vi "myRIO2.vi"() -> ()   [LabVIEW 2017]
uses:
  <vilib>/myRIO/Instrument Drivers/Onboard IO/DIO/typedefs/DIO Reference.ctl
  <vilib>/myRIO/Common/Instrument Driver Framework/Utilities/typedefs/myRIO Generic Hardware Reference.ctl
  <vilib>/myRIO/Common/Instrument Driver Framework/Utilities/typedefs/Hardware Version Enum.ctl
  <vilib>/myRIO/Common/Instrument Driver Framework/Utilities/typedefs/myRIO v1.0 Reference.ctl
  <vilib>/myRIO/Common/Instrument Driver Framework/Utilities/typedefs/Generic FPGA Reference.ctl
  <vilib>/myRIO/Common/Instrument Driver Framework/myRIO v1.0/DIO/typedefs/DIO Channels List.ctl
  <vilib>/myRIO/Common/Instrument Driver Framework/myRIO v1.0/DIO/typedefs/DIO Channels Enum.ctl
  <vilib>/userdefined/High Color/nirio_resource_hc.ctl
  <vilib>/Analysis/4window.llb/windowTd.ctl
  <vilib>/myRIO/Instrument Drivers/Onboard IO/UART/typedef/VISA Configuration.ctl
  <vilib>/myRIO/Common/Instrument Driver Framework/Utilities/vis/Is FPGA Ref Available.vi
  <vilib>/myRIO/Common/Instrument Driver Framework/myRIO v1.0/DIO/vis/myRIO v1.1 Open DIO.vi
  <vilib>/myRIO/Instrument Drivers/Onboard IO/DIO/vis/Write.vi
  <vilib>/myRIO/Instrument Drivers/Onboard IO/DIO/vis/Read.vi
  <vilib>/myRIO/Common/Instrument Driver Framework/Utilities/vis/Validate Channels.vi
  <vilib>/myRIO/Common/Instrument Driver Framework/myRIO v1.0/DIO/vis/myRIO v1.0 Reserve DIO.vi
  <vilib>/myRIO/Common/Instrument Driver Framework/myRIO v1.0/UART/vis/myRIO v1.0 Close UART.vi
  <vilib>/myRIO/Common/Instrument Driver Framework/myRIO v1.0/Resource Manager/vis/myRIO v1.0 Reserve Channel List.vi
  <vilib>/myRIO/Common/Instrument Driver Framework/myRIO v1.0/DIO/vis/myRIO v1.0 Build MUX Configuration DIO.vi
  <vilib>/myRIO/Common/Instrument Driver Framework/myRIO v1.0/Resource Manager/vis/myRIO v1.0 Reserve Channel.vi
  <vilib>/myRIO/Common/Instrument Driver Framework/myRIO v1.0/Resource Manager/vis/myRIO v1.0 Unreserve Channel.vi
  <vilib>/myRIO/Common/Instrument Driver Framework/myRIO v1.0/Resource Manager/vis/myRIO v1.0 Create Configuration List.vi
  <vilib>/myRIO/Common/Instrument Driver Framework/myRIO v1.0/Resource Manager/vis/myRIO v1.0 Build Mutex Name.vi
  <vilib>/Utility/VariantDataType/GetNumericInfo.vi
  <vilib>/Utility/error.llb/Error Cluster From Error Code.vi
  <vilib>/myRIO/Common/Instrument Driver Framework/myRIO v1.0/myRIO v1.1 Open.vi
  <vilib>/myRIO/Common/Instrument Driver Framework/Utilities/vis/IO Manager.vi
  <vilib>/myRIO/Common/Instrument Driver Framework/Utilities/vis/Configuration Manager.vi
  <vilib>/myRIO/Common/Instrument Driver Framework/myRIO v1.0/Resource Manager/vis/myRIO v1.0 Configure IO.vi
  <vilib>/myRIO/Common/Instrument Driver Framework/myRIO v1.0/myRIO v1.0 Close.vi
  <vilib>/myRIO/Common/Instrument Driver Framework/myRIO v1.0/DIO/vis/myRIO v1.0 Write DIO.vi
  <vilib>/FPGAPlugInAG/myRIO-1900/niLvFpga_Open_myRIO-1900.vi
  <vilib>/rvi/interface/common/dynamic/niFpgaDynamicAddResources.vi
  <vilib>/rvi/interface/common/niFpgaWaitOnOcc.vi
  <vilib>/rvi/errors/niLvFpgaAdjustHostInterfaceError.vi
  <vilib>/measure/maspectr.llb/FFT Power Spectrum and PSD for 1 Chan.vi
  <vilib>/FPGAPlugInAG/Dynamic/niLvFpga_Close_Dynamic.vi
  <vilib>/Instr/_visa.llb/VISA Configure Serial Port (Instr).vi
  <vilib>/myRIO/Common/Instrument Driver Framework/myRIO v1.0/DIO/vis/myRIO v1.0 Read DIO.vi
  <vilib>/Utility/file.llb/Write Delimited Spreadsheet (string).vi
  <vilib>/myRIO/Common/Instrument Driver Framework/Utilities/vis/FPGA Ref Manager.vi
  <vilib>/myRIO/Common/Instrument Driver Framework/myRIO v1.0/myRIO v1.0 Reset FPGA.vi
  <vilib>/myRIO/Common/Instrument Driver Framework/myRIO v1.0/IRQ/vis/myRIO v1.0 IRQ Info FGV.vi
  <vilib>/myRIO/Common/Instrument Driver Framework/myRIO v1.0/IRQ/vis/myRIO v1.0 Timer IRQ Info FGV.vi
  <vilib>/myRIO/Common/Instrument Driver Framework/myRIO v1.0/IRQ/vis/myRIO v1.0 ISR Agent.vi
  <vilib>/myRIO/Express VI/Onboard IO/DO/DO Express VI.xnode
  <vilib>/myRIO/Instrument Drivers/Onboard IO/DIO/vis/myRIO DIO Open.xnode
  <vilib>/rvi/interface/nirviOpenFPGA/nirviOpenFPGA.xnode
  drive-download-20180328T204708Z-001/Untitled Project 6/FPGA Bitfiles/UntitledProject6_FPGATarget_FPGA(1)_9+HZwm1Zn50.lvbitx
  FPGA (1).vi
  <vilib>/rvi/interface/nirviMethod/nirviMethod.xnode
  <vilib>/rvi/interface/nirviReadWriteControl/nirviReadWriteControl.xnode
  <vilib>/rvi/interface/nirviCloseFPGA/nirviCloseFPGA.xnode
  <vilib>/myRIO/Express VI/Onboard Devices/LED/LED Express VI.xnode
  <vilib>/myRIO/Express VI/Onboard IO/UART/UART Express VI.xnode
  <vilib>/myRIO/Express VI/Onboard IO/DI/DI Express VI.xnode
  <vilib>/myRIO/Express VI/Onboard Devices/Button/Button Express VI.xnode
  <vilib>/rvi/errors/niLvFpgaMergeErrorWithErrorCode.vi
  <vilib>/FPGAPlugInAG/Dynamic/niLvFpga_ReadFifo_Dynamic.vi
  <vilib>/FPGAPlugInAG/Dynamic/niLvFpga_ConfigureFifo_Dynamic.vi
  <vilib>/FPGAPlugInAG/Dynamic/niLvFpga_StartFifo_Dynamic.vi
  NiFpgaLv.dll
  <vilib>/rvi/interface/Simulation/niFpgaSimulationCallBeginRW.vi
  <vilib>/FPGAPlugInAG/Dynamic/niLvFpga_StopFifo_Dynamic.vi
  <vilib>/measure/NI_MAPro.lvlib
  <vilib>/myRIO/Instrument Drivers/Onboard IO/DIO/DIO.lvlib
  <vilib>/myRIO/Instrument Drivers/Onboard IO/UART/UART.lvlib
  <vilib>/myRIO/Instrument Drivers/Utilities/Utilities.lvlib
  <vilib>/Analysis/NI_AALPro.lvlib
panel:
  in  "Tab Control":enum32{"Logging  Data", "Amplitude Averaging"}(tab)
  out "Array 10":cluster{dbl, "y":dbl}[](array[cluster])
  out "Array 9":cluster{dbl, "y":dbl}[](array[cluster])
  out "Array 8":cluster{dbl, "y":dbl}[](array[cluster])
  out "Array 7":cluster{dbl, "y":dbl}[](array[cluster])
  out "Array 6":cluster{dbl, "y":dbl}[](array[cluster])
  out "element 2":cluster{dbl, "y":dbl}[](array[cluster])
  out "size":i32
  out "timed out?":bool
  out "# queue elements":i32
  out "Array 5":cluster{dbl, "y":dbl}[](array[cluster])
  in  "Array 4":cluster{dbl, "y":dbl}[](array[cluster])
  in  "Stop":bool
  out "Storage Device Failure":bool
  out "Data Queue Error":bool
  out "LinkIt Failure":bool
  out "DIO Failure":bool
  out "System Uptime":string
  out "Data Log Write Path":path
  out "Data Log":string[](array[string])
  out "D.L.H. Status":bool
  out "S.L.B. Status":bool
  out "D.L.B. Status":bool
  out "System Log Write Path":path
  out "System Log":string
  out "S.L.H. Status":bool
  out "Message Received":string
  out "M.R. Status":bool
  out "M.H. Status":bool
  out "LinkIt Response\nTimed Out 2":bool
  out "Time to Send \nMessage":dbl
  out "LinkIt Response\nTimed Out 3":bool
  out "LinkIt Response\nTimed Out 1":bool
  out "Pin 13 State":bool
  out "time to \nrespond":dbl
  out "Pin 11 State":bool
  out "Message to Send":string
  out "M.S. Status":bool
  out "?":i32(slide) scale=0.1..100.0
  out "S.L. Status":bool
  out "?":bool
  out "?":bool
  out "?":bool
  out "?":bool
  in  "Array 3":string[](array[string])
  out "Initialisation \nsuccessfull":bool
  in  "Min Frequency":dbl
  in  "Min Amplitude":dbl=0.001 format="%#_13g"
  out "Filtered Data Points":cluster{"X":dbl, "Y":dbl}[](graph)
  in  "averaging parameters":T1={"averaging mode"=enum."No averaging", "weighting mode"=enum."Exponential", "number of averages"=10} {"number of averages" min=1}
  out "Input Waveform":waveform(dbl)(graph)
  out "Power Spectrum":cluster{"f0":dbl, "df":dbl, "magnitude":dbl[]}(graph)
  out "error out":errorcluster
  out "Timed Out?":bool
  out "Maximum freq(Hz)":dbl
  out "Sampling freq(Hz)":dbl
  in  "Timeout (ms) 2":i32
  in  "No of Elements 2":u32=5000
  out "Element Read 2":i32
  out "Elements Remaining 2":u32
  out "Element Read":i32
  out "Current loop timing(ms)":u32
  in  "Count(uSec)":u32=16
  in  "Timeout (ms)":i32
  in  "No of Elements":u32
  out "Elements Remaining":u32
  in  "Requested Depth":u32=10000
  out "Actual Depth":u32=16384
  # "Project 2h - Version 1\nmyRIO1 Front Panel"
  # "FIFO configure"
  # "FPGA parameters"
  # "RT Loop Status"
  # "Signal Strength"
  # "Power Spectrum Options"
  # "Data point FIltering Options"
  # "FIFO Read"
  # "Outer"
  # "Inner"
  # "Rio \nDisplay"
  # "Elements to Read"
  # "Time out (ms)"
  # "Loop parameters"
  # "Elements Remaining"
  # "Elements Read"
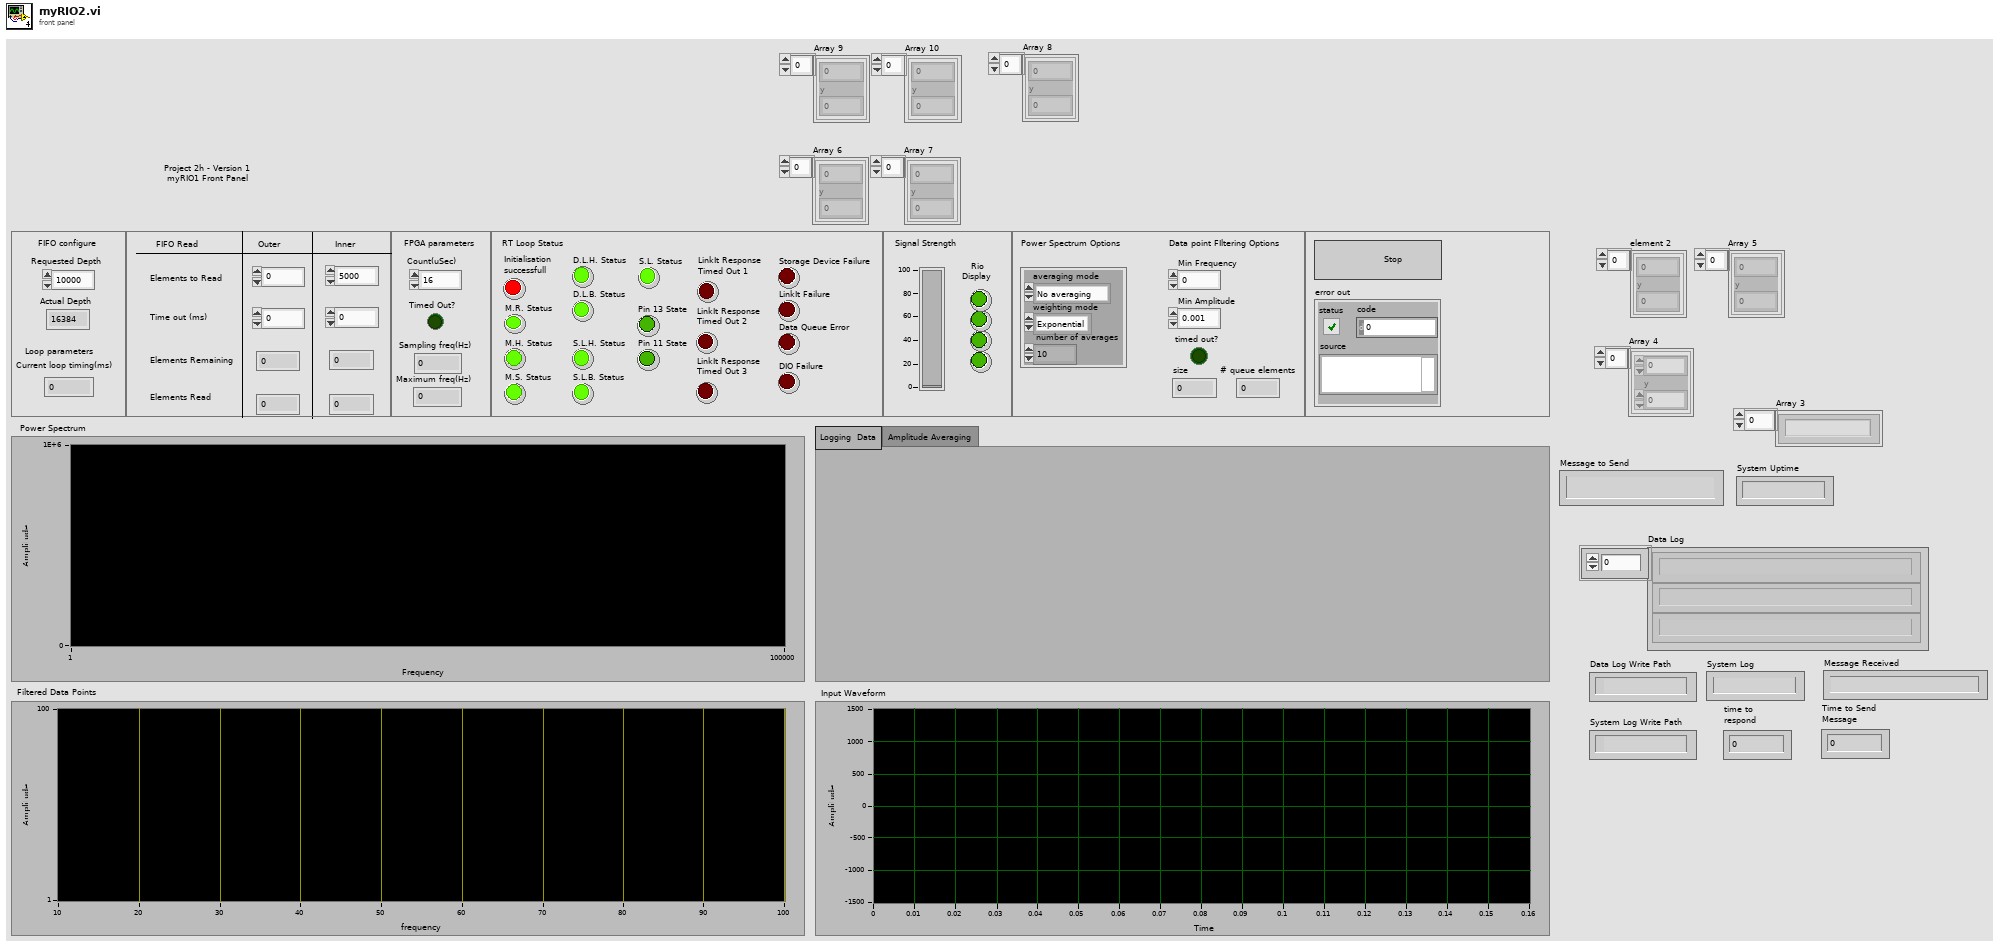
[diagram p1: front panel]
types:
  T1 = cluster{"averaging mode":enum16{"No averaging", "Vector averaging", "RMS averaging", "Peak hold"}, "weighting mode":enum16{"Linear", "Exponential"}, "number of averages":u32}
  T2 = cluster{string, string, string, string, string, string, string, string, string, string}
  T3 = typedef "DIO.lvlib/DIO Reference.ctl" = cluster{"myRIO Reference":T4, "DIO Channels List":T8}
  T4 = typedef "myRIO Generic Hardware Reference.ctl" = cluster{"myRIO Model":T5, "myRIO Hardware Reference":T6}
  T5 = typedef "Hardware Version Enum.ctl" = enum16{"Unknown", "myRIO-1900", "myRIO-1950", "roboRIO", "NI ELVIS RIO CM"}
  T6 = typedef "myRIO v1.0 Reference.ctl" = cluster{"Generic FPGA Reference":T7, "Allow multiple opens":bool}
  T7 = typedef "Generic FPGA Reference.ctl" = refnum<k20>
  T8 = typedef "DIO Channels List.ctl" = T9[]
  T9 = typedef "DIO Channels Enum.ctl" = enum16{"Not Connected", "C/DIO0", "C/DIO1", "C/DIO2", "C/DIO3", "C/DIO4", "C/DIO5", "C/DIO6", "C/DIO7", "A/DIO0", "A/DIO1", "A/DIO2", "A/DIO3", "A/DIO4", "A/DIO5", "A/DIO6", "A/DIO7", "A/DIO8", "A/DIO9", "A/DIO10", "A/DIO11", "A/DIO12", "A/DIO13", "A/DIO14", "A/DIO15", "B/DIO0", "B/DIO1", "B/DIO2", "B/DIO3", "B/DIO4", "B/DIO5", "B/DIO6", "B/DIO7", "B/DIO8", "B/DIO9", "B/DIO10", "B/DIO11", "B/DIO12", "B/DIO13", "B/DIO14", "B/DIO15", "LED0", "LED1", "LED2", "LED3", "Button0", "DIO/DIO0", "DIO/DIO1", "DIO/DIO2", "DIO/DIO3", "DIO/DIO4", "DIO/DIO5", "DIO/DIO6", "DIO/DIO7", "DIO/DIO8", "DIO/DIO9", "SPI/CS0", "SPI/CS1", "SPI/CS2", "SPI/CS3", "LED RADIO (Green)", "LED RADIO (Red)", "LED COMM (Green)", "LED COMM (Red)", "LED MODE (Green)", "LED MODE (Red)"}
  T10 = typedef "nirio_resource_hc.ctl" = tag
  T11 = typedef "UART.lvlib/VISA Configuration.ctl" = cluster{"baud rate (9600)":u32, "data bits (8)":u16, "parity (0:none)":enum16{"None", "Odd", "Even", "Mark", "Space"}, "stop bits (10: 1 bit)":u16, "flow control (0:none)":u16, "termination char\n(0xA = '\\n' = LF) ":u8, "Enable Termination\nChar (T)":bool, "timeout (10sec)":u32}
  T12 = enum16{"open", "replace", "create", "open or create", "replace or create", "replace or create with confirmation"}
  T13 = typedef "NI_AALPro.lvlib/windowTd.ctl" = u32
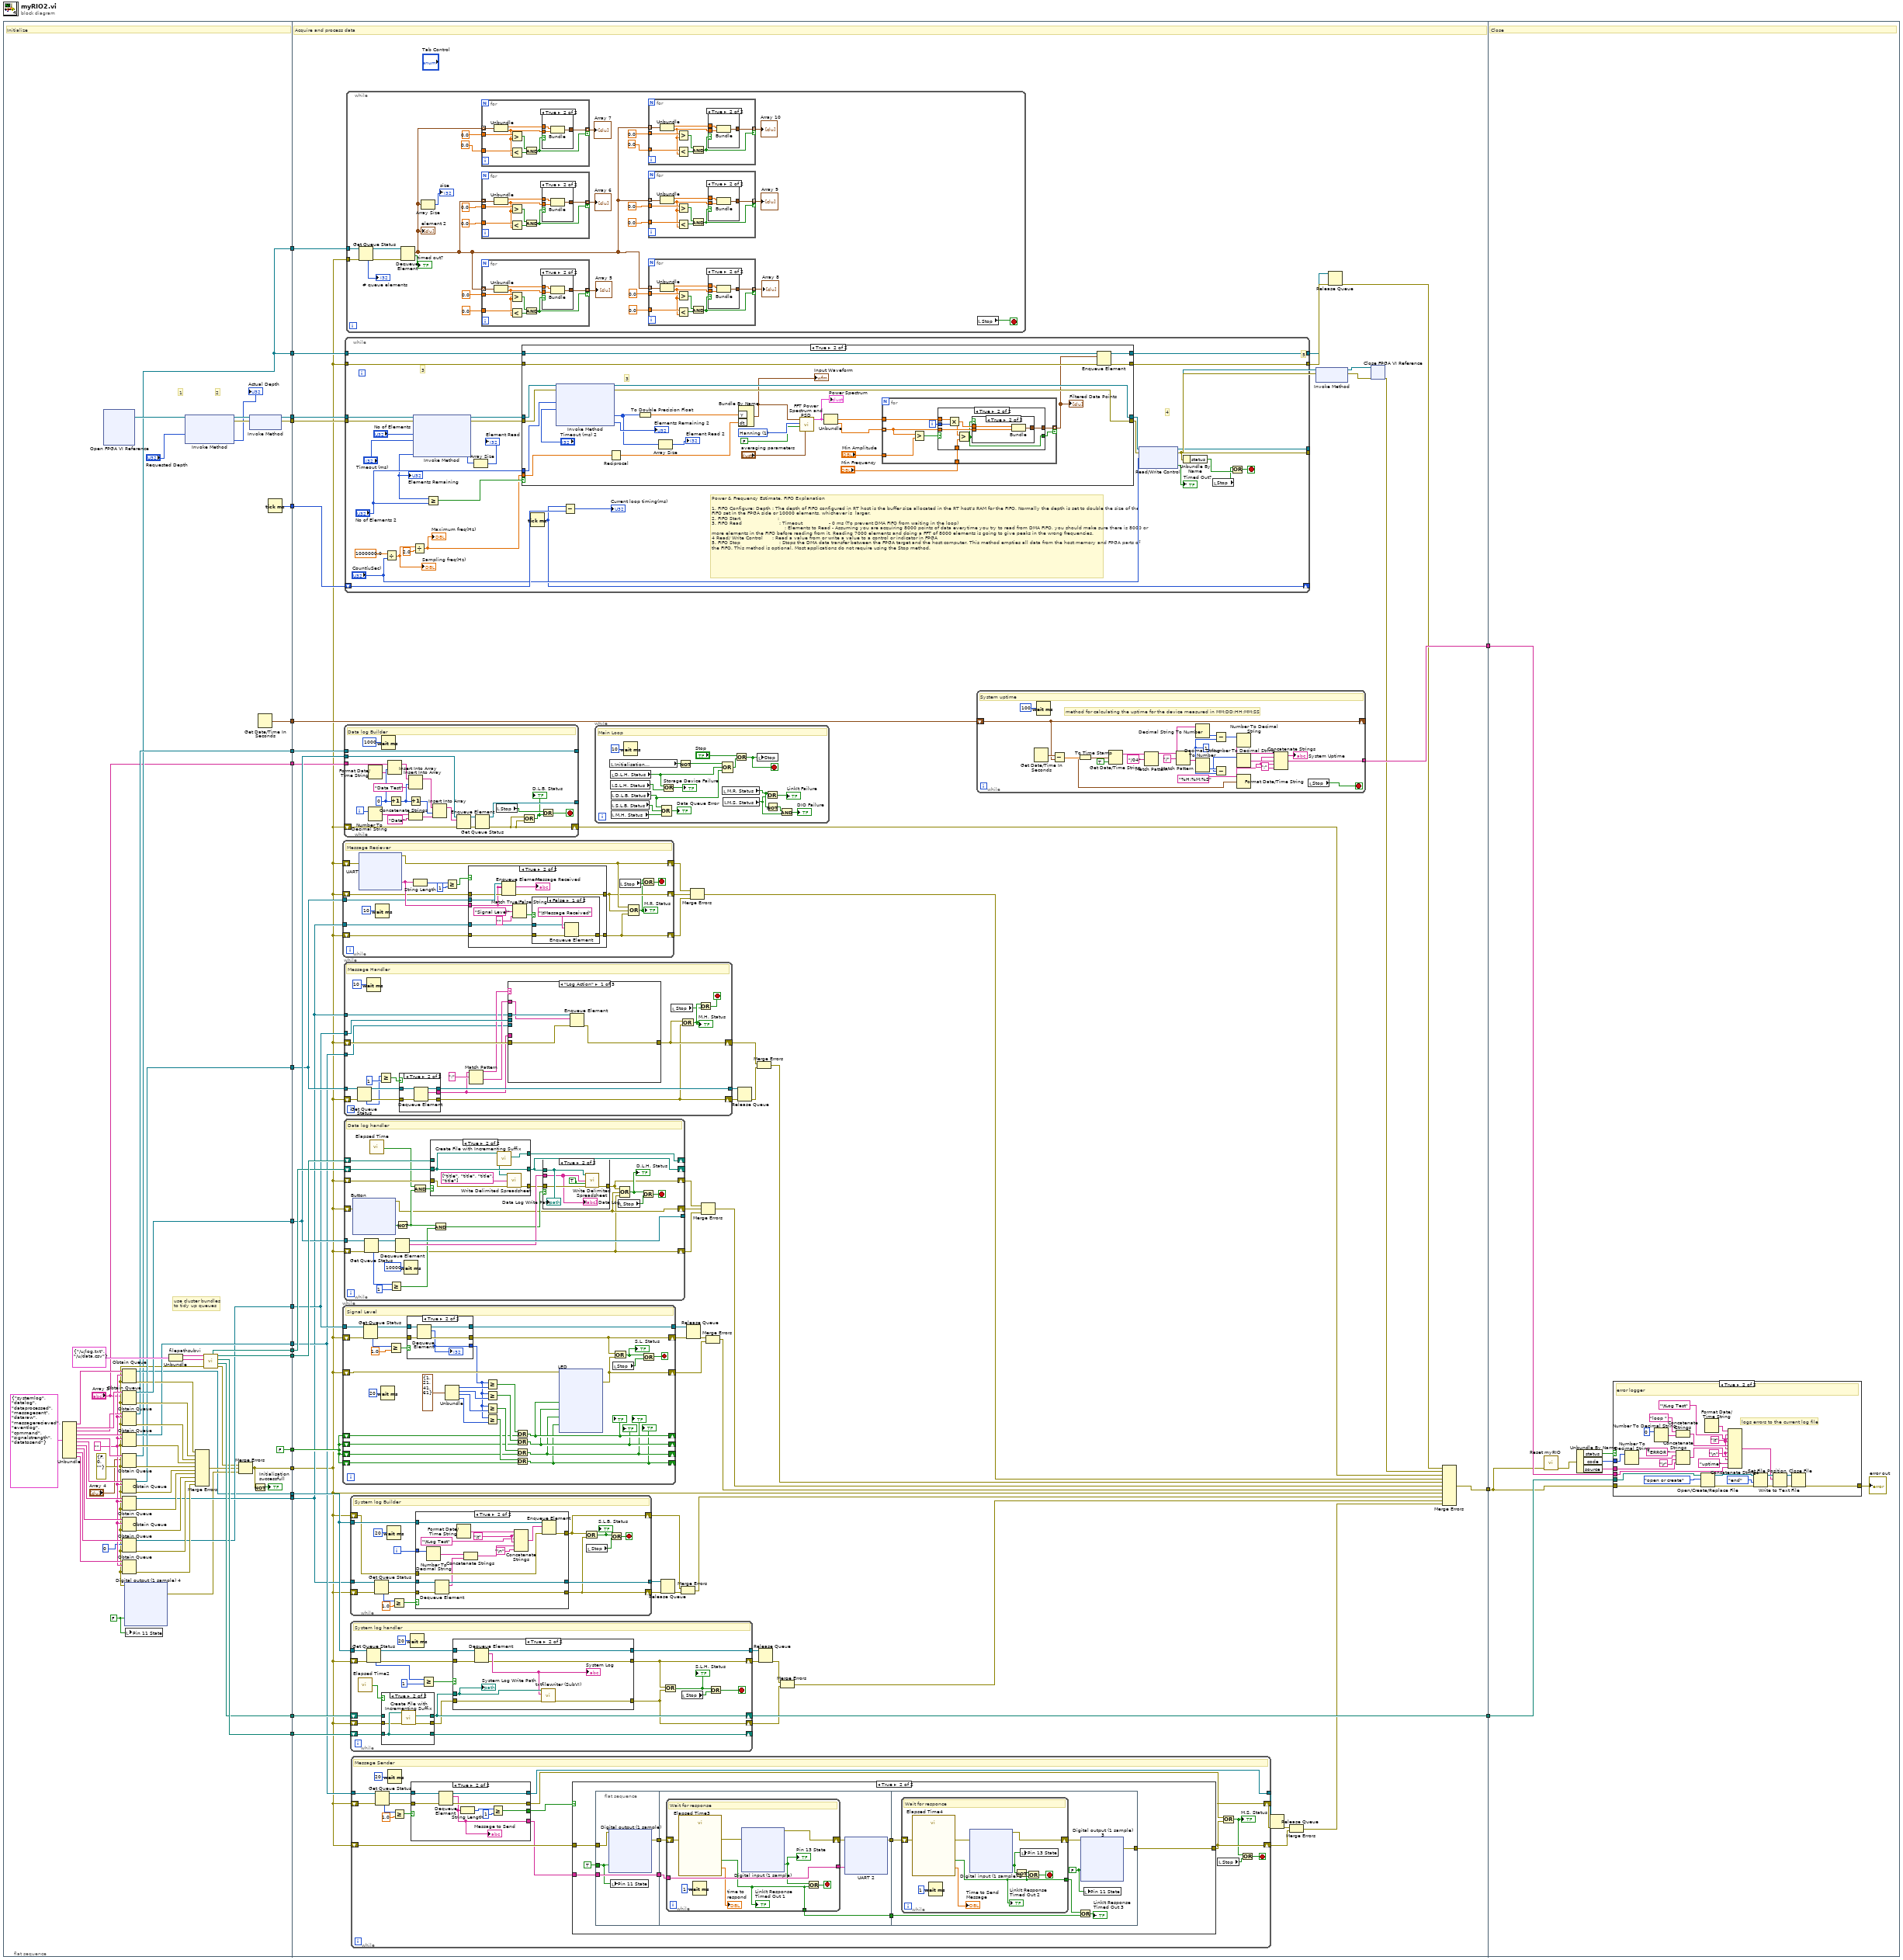
[diagram p0: block diagram]
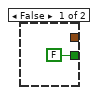
[diagram p9: hidden frame]
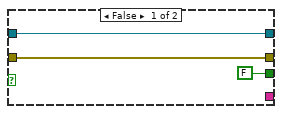
[diagram p12: hidden frame]
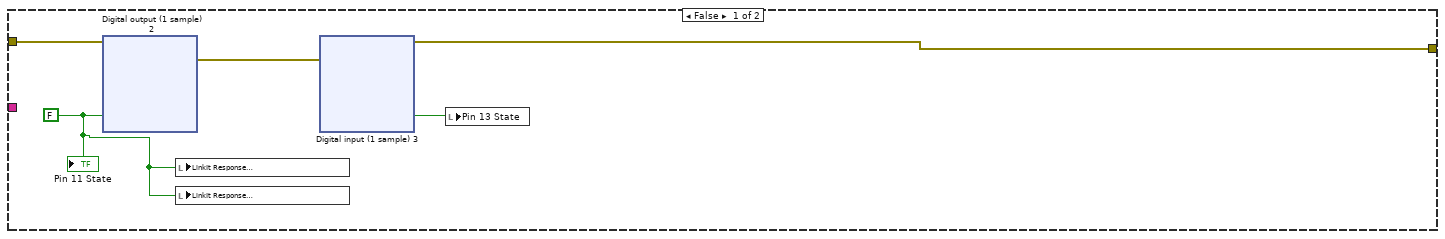
[diagram p13: hidden frame]
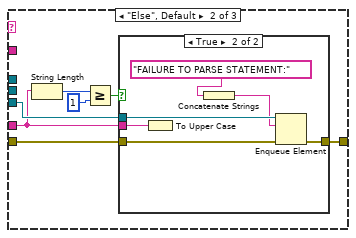
[diagram p15: hidden frame]
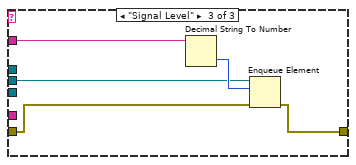
[diagram p17: hidden frame]
diagram:
  n1 = flat-sequence {
    tunnel: [w79] -> w23
    tunnel: [w70] -> w22
    tunnel: [w37] -> w21
    tunnel: [w69] -> w20
    tunnel: [w68] -> w19
    tunnel: [w35] -> w18
    tunnel: ["Array 3"] -> w17
    tunnel: [w36] -> w16
    tunnel: [w52] -> w15
    tunnel: [w51] -> w14
    tunnel: [w50] -> w13
    tunnel: [w49] -> w12
    tunnel: [w47] -> w11
    tunnel: [w46] -> w10
    tunnel: [FALSE] -> w9
    tunnel: [w29] -> w5
    tunnel: [w28] -> w4
    tunnel: [w27] -> w3
    tunnel: [w25] -> w2
    tunnel: [w25] -> w1
    tunnel: [w180] -> w8
    tunnel: w23 -> [w179]
    tunnel: w22 -> [w176]
    tunnel: w21 -> [w119]
    tunnel: w20 -> [w178]
    tunnel: w19 -> [w177]
    tunnel: w18 -> [w169]
    tunnel: w17 -> [w175]
    tunnel: w16 -> [w174]
    tunnel: w15 -> [w173]
    tunnel: w14 -> [w172]
    tunnel: [w171] -> w7
    tunnel: w13 -> [w170]
    tunnel: w12 -> [w141]
    tunnel: w11 -> [w131]
    tunnel: w10 -> [w144]
    tunnel: w9 -> [w166]
    tunnel: [w130] -> w6
    tunnel: w5 -> [w123]
    tunnel: w4 -> [w122]
    tunnel: w3 -> [w121]
    tunnel: w2 -> [w120]
    tunnel: w1 -> [w118]
    tunnel: w8 -> [w1064]
    tunnel: w7 -> [w1062]
    tunnel: w6 -> [w1061]
    frame #0 {
      w40 = FALSE
      w48 = ""
      w39 = errorcluster {"status"=FALSE, "code"=0, "source"=""} ("error in (no error)")
      # "2"
      # "1"
      # "use cluster bundles\nto tidy up queues"
      # "Initialize"
      n2 = Unbundle(T2 {"systemlog", "datalog", "dataprocessed", "messagesent", "dataraw", "messagerecieved", "eventlog", "command", "signalstrength", "datatosend"}) -> (w75:string, w74:string, w73:string, w72:string, w71:string, w62:string, w60:string, w59:string, w58:string, w57:string)
      n3 = xnode "Open FPGA VI Reference"() -> ("FPGA VI Reference Out"=w30:refnum<k20>)  [unwired: 2 in, 1 out]
      n4 = Obtain Queue(name (unnamed)=w75, element data type=w48, error in (no error)=w39) -> (queue out=w35:refnum<queue>, error out=w67:errorcluster)  [unwired: 2 in, 1 out]
      n5 = Obtain Queue(name (unnamed)=w74, element data type="Array 3", error in (no error)=w39) -> (queue out=w70:refnum<queue>, error out=w66:errorcluster)  [unwired: 2 in, 1 out]
      n6 = Obtain Queue(name (unnamed)=w73, element data type=w48, error in (no error)=w39) -> (queue out=w36:refnum<queue>, error out=w65:errorcluster)  [unwired: 2 in, 1 out]
      n7 = Obtain Queue(name (unnamed)=w72, element data type=w48, error in (no error)=w39) -> (queue out=w49:refnum<queue>, error out=w64:errorcluster)  [unwired: 2 in, 1 out]
      n8 = Obtain Queue(name (unnamed)=w71, element data type="Array 4", error in (no error)=w39) -> (queue out=w25:refnum<queue>, error out=w63:errorcluster)  [unwired: 2 in, 1 out]
      n9 = Obtain Queue(name (unnamed)=w62, element data type=w48, error in (no error)=w39) -> (queue out=w50:refnum<queue>, error out=w61:errorcluster)  [unwired: 2 in, 1 out]
      n10 = Obtain Queue(name (unnamed)=w60, element data type=w48, error in (no error)=w39) -> (queue out=w47:refnum<queue>, error out=w56:errorcluster)  [unwired: 2 in, 1 out]
      n11 = Obtain Queue(name (unnamed)=w59, element data type=w48, error in (no error)=w39) -> (error out=w55:errorcluster)  [unwired: 2 in, 2 out]
      n12 = Obtain Queue(name (unnamed)=w58, element data type=0, error in (no error)=w39) -> (queue out=w46:refnum<queue>, error out=w54:errorcluster)  [unwired: 2 in, 1 out]
      n13 = Obtain Queue(name (unnamed)=w57, element data type=w48, error in (no error)=w39) -> (error out=w53:errorcluster)  [unwired: 2 in, 2 out]
      n14 = xnode ("Digital output (1 sample) 4")("A/DIO0 (Pin 11)"=w40, "error in (no error)"=w39) -> ("error out"=w38:errorcluster)
      n15 = local write "Pin 11 State"(w40) -> ()
      n16 = Unbundle(cluster{string, string} {"/u/log.txt", "/u/data.csv"}) -> (w77:string, w76:string)
      n17 = xnode "Invoke Method"("FPGA VI Reference In"=w30, "Requested Depth"="Requested Depth") -> ("FPGA VI Reference Out"=w33:refnum<k20>, "error out"=w34:errorcluster, "Actual Depth"=→"Actual Depth":u32)  [unwired: 1 in]
      n18 = Merge Errors(w67, w66, w65, w64, w63, w61, w56, w55, w54, w53) -> (w42:errorcluster)
      n19 = call "filepathsubvi.vi"("error in (no error)"=w39, "String"=w76, "String 2"=w77) -> ("error out"=w41:errorcluster, "actual path"=w51:path, "Path"=w52:path, "actual path 2"=w69:path, "Path 2"=w68:path)  [unwired: 4 in]
      n20 = Merge Errors(w41, w42, w38) -> (w37:errorcluster)
      n21 = xnode "Invoke Method"("FPGA VI Reference In"=w33, "error in"=w34) -> ("FPGA VI Reference Out"=w28:refnum<k20>, "error out"=w27:errorcluster)
      n22 = Not(x=w37) -> (.not. x?=→"Initialisation \nsuccessfull":bool)
      n23 = Get Date/Time In Seconds() -> (seconds since 1Jan1904=w79:timestamp)
      n24 = Tick Count (ms)() -> (millisecond timer value=w29:u32)
    }
    frame #1 {
      # "5"
      # "Acquire and process data"
      n25 = while {
        shift-right: [w795] -> w151
        shift-left: w119 -> [w807]
        tunnel: w170 -> [w799]
        shift-right: [w794] -> w150
        shift-left: w119 -> [w798]
        shift-right: [w793] -> w149
        shift-left: w119 -> [w797]
        tunnel: w131 -> [w796]
        stop <- w804 stop-if-true
        # "Message Reciever"
        n26 = xnode "UART"("error in (no error)"=w807) -> ("Characters Read"=w800:string, "error out"=w795:errorcluster)
        n27 = Wait (ms)(milliseconds to wait=u32 10) -> ()  [unwired: 1 out]
        n28 = String Length(string=w800) -> (length=w802:i32)
        n29 = Greater Or Equal?(x=w802, y=1) -> (x >= y?=w803:bool)
        n30 = case shown="True" w803 {
          tunnel: w800 -> [_ w813]
          tunnel: w799 -> [_ w819]
          tunnel: w798 -> [w809 w818]
          tunnel: [w809 w817] -> w794
          tunnel: [w808 w816] -> w793
          tunnel: w797 -> [w808 w815]
          tunnel: w796 -> [_ w814]
          frame False {
          }
          frame True {
            n31 = Enqueue Element(queue=w819, element=w813, error in (no error)=w818) -> (error out=w817:errorcluster)  [unwired: 1 in, 2 out]
            n32 = Match True/False String(2:"" ("false string"), 3:"Signal Level" ("true string"), 4:w813) -> (0:w811:bool)  [unwired: 1 out]
            n33 = case shown="False" w811 {
              tunnel: [w822 w824] -> w816
              tunnel: w815 -> [w821 w824]
              tunnel: w814 -> [w820 _]
              frame False {
                n34 = Enqueue Element(queue=w820, element="\tMessage Received", error in (no error)=w821) -> (error out=w822:errorcluster)  [unwired: 1 in, 2 out]
              }
              frame True {
              }
            }
            "Message Received" <- w813
          }
        }
        n35 = local read "Stop"() -> (w805:bool)
        n36 = Compound Arithmetic op=OR(w795, w794, w793) -> (w792:bool)
        "M.R. Status" <- w792
        n37 = Or(x=w792, y=w805) -> (x .or. y?=w804:bool)
      }
      n38 = while {
        shift-right: [w365] -> w163
        shift-left: w119 -> [w376]
        shift-right: [w364] -> w154
        shift-left: w119 -> [w392]
        shift-right: [w369] -> _
        shift-left: w166 -> [w387]
        shift-right: [w368] -> _
        shift-left: w166 -> [w386]
        shift-right: [w367] -> _
        shift-left: w166 -> [w385]
        shift-right: [w366] -> _
        shift-left: w166 -> [w384]
        tunnel: w144 -> [w377]
        tunnel: [w375] -> w162
        stop <- w362 stop-if-true
        # "Signal Level"
        n39 = Get Queue Status(queue=w377, error in (no error)=w376) -> (queue out=w381:refnum<queue>, error out=w382:errorcluster, # elements in queue=w379:i32)  [unwired: 1 in, 5 out]
        n40 = Wait (ms)(milliseconds to wait=u32 20) -> ()  [unwired: 1 out]
        n41 = Greater Or Equal?(x=w379, y=1.0) -> (x >= y?=w380:bool)
        n42 = case shown="True" w380 {
          tunnel: w381 -> [w394 w399]
          tunnel: w382 -> [w393 w398]
          tunnel: [w394 w397] -> w375
          tunnel: [_ w395] -> w360
          tunnel: [w393 w396] -> w365
          frame False {
          }
          frame True {
            n43 = Dequeue Element(queue=w399, error in (no error)=w398) -> (queue out=w397:refnum<queue>, element=w395:i32, error out=w396:errorcluster)  [unwired: 1 in, 1 out]
            "?" <- w395
          }
        }
        n44 = Unbundle(cluster{i32, i32, i32, i32} {1, 21, 41, 61}) -> (w373:i32, w372:i32, w371:i32, w370:i32)
        n45 = Greater Or Equal?(x=w360, y=w373) -> (x >= y?=w391:bool)
        n46 = Greater Or Equal?(x=w360, y=w372) -> (x >= y?=w390:bool)
        n47 = Greater Or Equal?(x=w360, y=w371) -> (x >= y?=w389:bool)
        n48 = Greater Or Equal?(x=w360, y=w370) -> (x >= y?=w388:bool)
        n49 = Or(x=w391, y=w387) -> (x .or. y?=w369:bool)
        "?" <- w369
        n50 = Or(x=w390, y=w386) -> (x .or. y?=w368:bool)
        "?" <- w368
        n51 = Or(x=w389, y=w385) -> (x .or. y?=w367:bool)
        "?" <- w367
        n52 = Or(x=w388, y=w384) -> (x .or. y?=w366:bool)
        "?" <- w366
        n53 = xnode "LED"("61+"=w369, "41-60"=w368, "21-40"=w367, "1-20"=w366, "error in (no error)"=w392) -> ("error out"=w364:errorcluster)
        n54 = local read "Stop"() -> (w363:bool)
        n55 = Compound Arithmetic op=OR(w365, w364) -> (w361:bool)
        "S.L. Status" <- w361
        n56 = Or(x=w361, y=w363) -> (x .or. y?=w362:bool)
      }
      n57 = while {
        tunnel: [w760] -> w145
        tunnel: w170 -> [w759]
        shift-right: [w748] -> w146
        shift-left: w119 -> [w746]
        shift-right: [w753] -> w147
        shift-left: w119 -> [w757]
        tunnel: w144 -> [w756]
        tunnel: w141 -> [w749]
        tunnel: w131 -> [w740]
        stop <- w752 stop-if-true
        # "Message Handler"
        n58 = Get Queue Status(queue=w759, error in (no error)=w746) -> (queue out=w747:refnum<queue>, error out=w745:errorcluster, # elements in queue=w742:i32)  [unwired: 1 in, 5 out]
        n59 = Wait (ms)(milliseconds to wait=u32 10) -> ()  [unwired: 1 out]
        n60 = Greater Or Equal?(x=w742, y=1) -> (x >= y?=w743:bool)
        n61 = case shown="True" w743 {
          tunnel: [w763 w768] -> w760
          tunnel: [_ w767] -> w741
          tunnel: [w762 w766] -> w748
          tunnel: w747 -> [w763 w765]
          tunnel: w745 -> [w762 w764]
          frame False {
          }
          frame True {
            n62 = Dequeue Element(queue=w765, error in (no error)=w764) -> (queue out=w768:refnum<queue>, element=w767:string, error out=w766:errorcluster)  [unwired: 1 in, 1 out]
          }
        }
        n63 = Match Pattern(string=w741, regular expression=":") -> (before substring=w754:string, after substring=w755:string)  [unwired: 1 in, 2 out]
        n64 = case shown="\"Log Action\"" w754 {
          tunnel: w755 -> [w769 _ w790]
          tunnel: w757 -> [w772 w778 w789]
          tunnel: [w770 w777 w788] -> w753
          tunnel: w756 -> [_ _ w787]
          tunnel: w741 -> [_ w774 _]
          tunnel: w749 -> [_ w779 _]
          tunnel: w740 -> [w771 _ _]
          frame "Log Action" {
            n65 = Enqueue Element(queue=w771, element=w769, error in (no error)=w772) -> (error out=w770:errorcluster)  [unwired: 1 in, 2 out]
          }
          frame "Else", Default {
            n66 = String Length(string=w774) -> (length=w775:i32)
            n67 = Greater Or Equal?(x=w775, y=1) -> (x >= y?=w773:bool)
            n68 = case shown="True" w773 {
              tunnel: w779 -> [_ w786]
              tunnel: w778 -> [w780 w785]
              tunnel: [w780 w784] -> w777
              tunnel: w774 -> [_ w782]
              frame False {
              }
              frame True {
                n69 = To Upper Case(1:w782) -> ()  [unwired: 1 out]
                n70 = Concatenate Strings("FAILURE TO PARSE STATEMENT:") -> (w783:string)
                n71 = Enqueue Element(queue=w786, element=w783, error in (no error)=w785) -> (error out=w784:errorcluster)  [unwired: 1 in, 2 out]
              }
            }
          }
          frame "Signal Level" {
            n72 = Decimal String To Number(string=w790) -> (number=w791:i32)  [unwired: 2 in, 1 out]
            n73 = Enqueue Element(queue=w787, element=w791, error in (no error)=w789) -> (error out=w788:errorcluster)  [unwired: 1 in, 2 out]
          }
        }
        n74 = local read "Stop"() -> (w750:bool)
        n75 = Compound Arithmetic op=OR(w753, w748) -> (w751:bool)
        "M.H. Status" <- w751
        n76 = Or(x=w751, y=w750) -> (x .or. y?=w752:bool)
      }
      n77 = while {
        shift-right: [w959] -> w142
        shift-left: w119 -> [w955]
        tunnel: w176 -> [w967]
        tunnel: [w965] -> _
        shift-right: [w954] -> _
        shift-left: w177 -> [w953]
        shift-right: [w950] -> _
        shift-left: w178 -> [w951]
        shift-right: [w941] -> w148
        shift-left: w119 -> [w966]
        shift-right: [w942] -> w143
        shift-left: w119 -> [w943]
        stop <- w956 stop-if-true
        # "Data log handler"
        n78 = xnode "Button"("error in (no error)"=w943) -> ("Value"=w949:bool, "error out"=w942:errorcluster)
        n79 = Get Queue Status(queue=w967, error in (no error)=w966) -> (queue out=w964:refnum<queue>, error out=w963:errorcluster, # elements in queue=w962:i32)  [unwired: 1 in, 5 out]
        n80 = call "Elapsed Time"() -> ("Time has Elapsed"=w948:bool)  [unwired: 12 in, 7 out]
        n81 = Greater Or Equal?(x=w962, y=1) -> (x >= y?=w945:bool)
        n82 = Dequeue Element(queue=w964, error in (no error)=w963) -> (queue out=w965:refnum<queue>, element=w957:string[], error out=w941:errorcluster)  [unwired: 1 in, 1 out]
        n83 = Not(x=w949) -> (.not. x?=w946:bool)
        n84 = Wait (ms)(milliseconds to wait=u32 10000) -> ()  [unwired: 1 out]
        n85 = And(x=w948, y=w946) -> (x .and. y?=w947:bool)
        n86 = case shown="True" w947 {
          tunnel: w955 -> [w1005 w1011]
          tunnel: [w1006 w1008] -> w954
          tunnel: w953 -> [w1006 w1008]
          tunnel: [w1005 w1010] -> w952
          tunnel: w951 -> [w1004 _]
          tunnel: [w1004 w1007] -> w950
          frame False {
          }
          frame True {
            n87 = call <vilib>:"Create File with Incrementing Suffix.vi"("file path"=w1008) -> ("actual path"=w1007:path)  [unwired: 8 in, 2 out]
            n88 = call-poly <vilib>:"Write Delimited Spreadsheet.vi"("file path (dialog if empty)"=w1007, "1D data"=string[] ["title", "title", "title", "title"], "error in (no error)"=w1011) -> ("error out"=w1010:errorcluster)  [unwired: 11 in, 1 out]
          }
        }
        n89 = And(x=w946, y=w945) -> (x .and. y?=w944:bool)
        n90 = case shown="True" w944 {
          tunnel: w952 -> [w1012 w1016]
          tunnel: w954 -> [_ w1017]
          tunnel: [w1012 w1015] -> w959
          tunnel: w957 -> [_ w1013]
          frame False {
          }
          frame True {
            n91 = call-poly <vilib>:"Write Delimited Spreadsheet.vi"("file path (dialog if empty)"=w1017, "1D data"=w1013, "append to file? (new file:F)"=TRUE, "error in (no error)"=w1016) -> ("error out"=w1015:errorcluster)  [unwired: 10 in, 1 out]
            "Data Log Write Path" <- w1017
            "Data Log" <- w1013
          }
        }
        n92 = local read "Stop"() -> (w958:bool)
        n93 = Compound Arithmetic op=OR(w959, w942, w941) -> (w960:bool)
        "D.L.H. Status" <- w960
        n94 = Or(x=w960, y=w958) -> (x .or. y?=w956:bool)
      }
      n95 = while {
        tunnel: w176 -> [w903]
        tunnel: [w900] -> _
        tunnel: [w884] -> _
        tunnel: w174 -> [w884]
        tunnel: w175 -> [w883]
        shift-right: [w882] -> w139
        shift-left: w119 -> [w899]
        i -> [w887]
        stop <- w886 stop-if-true
        w895 = 0
        # "Data log Builder"
        n96 = Format Date/Time String() -> (date/time string=w892:string)  [unwired: 3 in]
        n97 = Number To Decimal String(number=w887) -> (decimal integer string=w890:string)  [unwired: 1 in]
        n98 = Wait (ms)(milliseconds to wait=u32 1000) -> ()  [unwired: 1 out]
        n99 = Insert Into Array(array=w883, index=w895, new element=w892) -> (w898:string[])
        n100 = Increment(x=w895) -> (x+1=w894:i32)
        n101 = Concatenate Strings(w890, "Data") -> (w888:string)
        n102 = Insert Into Array(array=w898, index=w894, new element="Data Test" ("text")) -> (w897:string[])
        n103 = Increment(x=w894) -> (x+1=w893:i32)
        n104 = Insert Into Array(array=w897, index=w893, new element=w888) -> (w896:string[])
        n105 = Enqueue Element(queue=w903, element=w896, error in (no error)=w899) -> (queue out=w901:refnum<queue>, error out=w902:errorcluster)  [unwired: 1 in, 1 out]
        n106 = Get Queue Status(queue=w901, error in (no error)=w902) -> (queue out=w900:refnum<queue>, error out=w882:errorcluster)  [unwired: 1 in, 6 out]
        n107 = local read "Stop"() -> (w885:bool)
        n108 = Compound Arithmetic op=OR(w882, w882) -> (w881:bool)
        "D.L.B. Status" <- w881
        n109 = Or(x=w885, y=w881) -> (x .or. y?=w886:bool)
      }
      n110 = while {
        tunnel: w122 -> [w310]
        tunnel: w121 -> [w309]
        tunnel: [w305] -> w124
        tunnel: [w288] -> w125
        shift-right: [w289] -> _
        shift-left: w123 -> [w303]
        tunnel: w120 -> [w286]
        tunnel: [w285] -> w128
        tunnel: w119 -> [w284]
        tunnel: [w283] -> w129
        stop <- w306 stop-if-true
        # "Power & Frequency Estimate. FIFO Explanation\n\n1. FIFO Configure: Depth : The depth of FIFO configured in RT host is the buffer size allocated in the RT host's RAM for the FIFO. Normally the depth is set to double the size of the FIFO set in the FPGA side or 10000 elements, whichever is  larger.\n2. FIFO Start                        :\n3. FIFO Read                        : Timeout                 - 0 ms (To prevent DMA FIFO from waiting in the loop) \n                                               : Elements to Read - Assuming you are acquiring 8000 points of data everytime you try to read from DMA FIFO, you should make sure there is 8000 or more elements in the FIFO before reading from it. Reading 7000 elements and doing a FFT of 8000 elements is going to give peaks in the wrong frequencies.\n4 Read/ Write Control      : Read a value from or write a value to a control or indicator in FPGA \n5. FIFO Stop                         : Stops the DMA data transfer between the FPGA target and the host computer. This method empties all data from the host memory and FPGA parts of the FIFO. This method is optional. Most applications do not require using the Stop method."
        # "4"
        # "3"
        n111 = Divide(x=1000000.0 ("y"), y="Count(uSec)") -> (x/y=w282:dbl)
        "Sampling freq(Hz)" <- w282
        n112 = Divide(x=w282, y=2.0) -> (x/y=w281:dbl)
        "Maximum freq(Hz)" <- w281
        n113 = xnode "Invoke Method"("FPGA VI Reference In"=w310, "error in"=w309, "Number of Elements"="No of Elements", "Timeout (ms)"="Timeout (ms)") -> ("FPGA VI Reference Out"=w297:refnum<k20>, "error out"=w296:errorcluster, "Data"=w301:i16[], "Elements Remaining"=w299:u32)
        "Elements Remaining" <- w299
        n114 = Greater Or Equal?(x=w299, y="No of Elements 2") -> (x >= y?=w298:bool)
        n115 = Array Size(array=w301) -> (size(s)=→"Element Read":i32)
        n116 = case shown="True" w298 {
          tunnel: "No of Elements 2" -> [_ w340]
          tunnel: w297 -> [w314 w339]
          tunnel: w296 -> [w313 w338]
          tunnel: [w314 w337] -> w295
          tunnel: [w313 w330] -> w294
          tunnel: w286 -> [w311 w327]
          tunnel: [w311 w326] -> w285
          tunnel: w284 -> [w312 w325]
          tunnel: [w312 w324] -> w283
          tunnel: w281 -> [_ w321]
          frame False {
          }
          frame True {
            w333 = T13 1 items=["Rectangle"=0, "Hanning"=1, "Hamming"=2, "Blackman-Harris"=3, "Exact Blackman"=4, "Blackman"=5, "Flat Top"=6, "4 Term B-Harris "=7, "7 Term B-Harris"=8, "Low Sidelobe"=9, "Blackman Nuttall"=11, "Triangle"=30, "Bartlett-Hanning"=31, "Bohman"=32, "Parzen"=33, "Welch"=34, "Kaiser"=60, "Dolph-Chebyshev"=61, "Gaussian"=62] ("window")
            # "3"
            n117 = xnode "Invoke Method"("FPGA VI Reference In"=w339, "error in"=w338, "Number of Elements"=w340, "Timeout (ms)"="Timeout (ms) 2") -> ("FPGA VI Reference Out"=w337:refnum<k20>, "error out"=w330:errorcluster, "Data"=w331:i16[], "Elements Remaining"=→"Elements Remaining 2":u32)
            n118 = Reciprocal(x=w321) -> (1/x=w329:dbl)
            n119 = To Double Precision Float(number=w331) -> (double precision float=w322:dbl[])
            n120 = Array Size(array=w331) -> (size(s)=→"Element Read 2":i32)
            n121 = Bundle By Name("Y"=w322, "dt"=w329) -> (w323:waveform(dbl))  [unwired: 1 in]
            "Input Waveform" <- w323
            n122 = call-poly <vilib>:"FFT Power Spectrum and PSD.vi"("averaging parameters"="averaging parameters", "dB On (F)"=FALSE, "window"=w333, "time signal"=w323) -> ("Power Spectrum / PSD"=w320:cluster{"f0":dbl, "df":dbl, "magnitude":dbl[]})  [unwired: 4 in, 3 out]
            "Power Spectrum" <- w320
            n123 = Unbundle(w320) -> ("df"=w319:dbl, "magnitude"=w316:dbl[])  [unwired: 1 out]
            n124 = for {
              tunnel: w316 -> [w346] mode=indexing
              tunnel: w319 -> [w348]
              tunnel: [w345] -> w315 mode=indexing if=w341
              tunnel: "Min Amplitude" -> [w344]
              tunnel: "Min Frequency" -> [w343]
              i -> [w347]
              n125 = Greater?(x=w346, y=w344) -> (0:w342:bool)
              n126 = case shown="True" w342 {
                tunnel: w348 -> [_ w356]
                tunnel: w347 -> [_ w353]
                tunnel: w346 -> [_ w354]
                tunnel: [_ w355] -> w345
                tunnel: w343 -> [_ w351]
                tunnel: [FALSE w350] -> w341
                frame False {
                }
                frame True {
                  n127 = Multiply(x=w356, y=w353) -> (x*y=w352:dbl)
                  n128 = Greater?(x=w352, y=w351) -> (0:w350:bool)
                  n129 = case shown="True" w350 {
                    tunnel: [_ w359] -> w355
                    tunnel: w352 -> [_ w358]
                    tunnel: w354 -> [_ w357]
                    frame False {
                    }
                    frame True {
                      n130 = Bundle(w358, "Numeric"=w357) -> (w359:cluster{dbl, "Numeric":dbl})  [unwired: 1 in]
                    }
                  }
                }
              }
            }
            "Filtered Data Points" <- w315
            n131 = Enqueue Element(queue=w327, element=w315, error in (no error)=w325) -> (queue out=w326:refnum<queue>, error out=w324:errorcluster)  [unwired: 1 in, 1 out]
          }
        }
        n132 = Tick Count (ms)() -> (millisecond timer value=w289:u32)
        n133 = Subtract(x=w289, y=w303) -> (x-y=→"Current loop timing(ms)":u32)
        n134 = xnode "Read/Write Control"("FPGA VI Reference In"=w295, "error in"=w294, "Count(uSec)"="Count(uSec)") -> ("FPGA VI Reference Out"=w305:refnum<k20>, "error out"=w288:errorcluster, "Timed Out?"=→"Timed Out?":bool)
        n135 = Unbundle By Name(w288) -> ("status"=w287:bool)
        n136 = local read "Stop"() -> (w280:bool)
        n137 = Or(x=w280, y=w287) -> (x .or. y?=w306:bool)
      }
      n138 = while {
        tunnel: w118 -> [w205]
        tunnel: w119 -> [w203]
        stop <- w191 stop-if-true
        n139 = Get Queue Status(queue=w205, error in (no error)=w203) -> (queue out=w204:refnum<queue>, error out=w202:errorcluster, # elements in queue=→"# queue elements":i32)  [unwired: 1 in, 5 out]
        n140 = Dequeue Element(queue=w204, error in (no error)=w202) -> (element=w181:cluster{dbl, "y":dbl}[], timed out?=→"timed out?":bool)  [unwired: 1 in, 2 out]
        "element 2" <- w181
        n141 = Array Size(array=w181) -> (size(s)=→"size":i32)
        n142 = for {
          tunnel: w181 -> [w252] mode=indexing
          tunnel: 0.0 -> [w251]
          tunnel: 0.0 -> [w250]
          tunnel: [w245] -> w193 mode=indexing if=w244
          n143 = Unbundle(w252) -> (w247:dbl, "y"=w246:dbl)
          n144 = Greater?(x=w250, y=w246) -> (0:w249:bool)
          n145 = Less?(x=w251, y=w246) -> (x < y?=w248:bool)
          n146 = And(x=w249, y=w248) -> (x .and. y?=w244:bool)
          n147 = case shown="True" w244 {
            tunnel: w247 -> [_ w255]
            tunnel: w246 -> [_ w254]
            tunnel: [_ w253] -> w245
            frame False {
            }
            frame True {
              n148 = Bundle(w255, "y"=w254) -> (w253:cluster{dbl, "y":dbl})  [unwired: 1 in]
            }
          }
        }
        "Array 7" <- w193
        n149 = for {
          tunnel: w181 -> [w264] mode=indexing
          tunnel: 0.0 -> [w263]
          tunnel: 0.0 -> [w262]
          tunnel: [w257] -> w192 mode=indexing if=w256
          n150 = Unbundle(w264) -> (w259:dbl, "y"=w258:dbl)
          n151 = Greater?(x=w262, y=w258) -> (0:w261:bool)
          n152 = Less?(x=w263, y=w258) -> (x < y?=w260:bool)
          n153 = And(x=w261, y=w260) -> (x .and. y?=w256:bool)
          n154 = case shown="True" w256 {
            tunnel: w259 -> [_ w267]
            tunnel: w258 -> [_ w266]
            tunnel: [_ w265] -> w257
            frame False {
            }
            frame True {
              n155 = Bundle(w267, "y"=w266) -> (w265:cluster{dbl, "y":dbl})  [unwired: 1 in]
            }
          }
        }
        "Array 6" <- w192
        n156 = for {
          tunnel: w181 -> [w276] mode=indexing
          tunnel: 0.0 -> [w275]
          tunnel: 0.0 -> [w274]
          tunnel: [w269] -> w198 mode=indexing if=w268
          n157 = Unbundle(w276) -> (w271:dbl, "y"=w270:dbl)
          n158 = Greater?(x=w274, y=w270) -> (0:w273:bool)
          n159 = Less?(x=w275, y=w270) -> (x < y?=w272:bool)
          n160 = And(x=w273, y=w272) -> (x .and. y?=w268:bool)
          n161 = case shown="True" w268 {
            tunnel: w271 -> [_ w279]
            tunnel: w270 -> [_ w278]
            tunnel: [_ w277] -> w269
            frame False {
            }
            frame True {
              n162 = Bundle(w279, "y"=w278) -> (w277:cluster{dbl, "y":dbl})  [unwired: 1 in]
            }
          }
        }
        "Array 5" <- w198
        n163 = for {
          tunnel: w181 -> [w216] mode=indexing
          tunnel: 0.0 -> [w215]
          tunnel: 0.0 -> [w214]
          tunnel: [w209] -> w183 mode=indexing if=w208
          n164 = Unbundle(w216) -> (w211:dbl, "y"=w210:dbl)
          n165 = Greater?(x=w214, y=w210) -> (0:w213:bool)
          n166 = Less?(x=w215, y=w210) -> (x < y?=w212:bool)
          n167 = And(x=w213, y=w212) -> (x .and. y?=w208:bool)
          n168 = case shown="True" w208 {
            tunnel: w211 -> [_ w219]
            tunnel: w210 -> [_ w218]
            tunnel: [_ w217] -> w209
            frame False {
            }
            frame True {
              n169 = Bundle(w219, "y"=w218) -> (w217:cluster{dbl, "y":dbl})  [unwired: 1 in]
            }
          }
        }
        "Array 10" <- w183
        n170 = for {
          tunnel: w181 -> [w228] mode=indexing
          tunnel: 0.0 -> [w227]
          tunnel: 0.0 -> [w226]
          tunnel: [w221] -> w182 mode=indexing if=w220
          n171 = Unbundle(w228) -> (w223:dbl, "y"=w222:dbl)
          n172 = Greater?(x=w226, y=w222) -> (0:w225:bool)
          n173 = Less?(x=w227, y=w222) -> (x < y?=w224:bool)
          n174 = And(x=w225, y=w224) -> (x .and. y?=w220:bool)
          n175 = case shown="True" w220 {
            tunnel: w223 -> [_ w231]
            tunnel: w222 -> [_ w230]
            tunnel: [_ w229] -> w221
            frame False {
            }
            frame True {
              n176 = Bundle(w231, "y"=w230) -> (w229:cluster{dbl, "y":dbl})  [unwired: 1 in]
            }
          }
        }
        "Array 9" <- w182
        n177 = for {
          tunnel: w181 -> [w240] mode=indexing
          tunnel: 0.0 -> [w239]
          tunnel: 0.0 -> [w238]
          tunnel: [w233] -> w188 mode=indexing if=w232
          n178 = Unbundle(w240) -> (w235:dbl, "y"=w234:dbl)
          n179 = Greater?(x=w238, y=w234) -> (0:w237:bool)
          n180 = Less?(x=w239, y=w234) -> (x < y?=w236:bool)
          n181 = And(x=w237, y=w236) -> (x .and. y?=w232:bool)
          n182 = case shown="True" w232 {
            tunnel: w235 -> [_ w243]
            tunnel: w234 -> [_ w242]
            tunnel: [_ w241] -> w233
            frame False {
            }
            frame True {
              n183 = Bundle(w243, "y"=w242) -> (w241:cluster{dbl, "y":dbl})  [unwired: 1 in]
            }
          }
        }
        "Array 8" <- w188
        n184 = local read "Stop"() -> (w191:bool)
      }
      n185 = while {
        shift-right: [w908] -> w158
        shift-left: w119 -> [w909]
        tunnel: w131 -> [w914]
        tunnel: [w912] -> w168
        shift-right: [w907] -> w167
        shift-left: w119 -> [w913]
        tunnel: w169 -> [w910]
        i -> [w905]
        stop <- w919 stop-if-true
        # "System log Builder"
        n186 = Get Queue Status(queue=w914, error in (no error)=w913) -> (queue out=w916:refnum<queue>, error out=w915:errorcluster, # elements in queue=w918:i32)  [unwired: 1 in, 5 out]
        n187 = Wait (ms)(milliseconds to wait=u32 20) -> ()  [unwired: 1 out]
        n188 = Greater Or Equal?(x=w918, y=1.0) -> (x >= y?=w911:bool)
        n189 = case shown="True" w911 {
          tunnel: w916 -> [w923 w940]
          tunnel: w915 -> [w924 w939]
          tunnel: [w923 w938] -> w912
          tunnel: [w924 w937] -> w907
          tunnel: w905 -> [_ w930]
          tunnel: w910 -> [_ w929]
          tunnel: w909 -> [w922 w927]
          tunnel: [w922 w925] -> w908
          frame False {
          }
          frame True {
            w933 = "\t"
            n190 = Number To Decimal String(number=w930) -> (decimal integer string=w934:string)  [unwired: 1 in]
            n191 = Dequeue Element(queue=w940, error in (no error)=w939) -> (queue out=w938:refnum<queue>, element=w926:string, error out=w937:errorcluster)  [unwired: 1 in, 1 out]
            n192 = Format Date/Time String() -> (date/time string=w935:string)  [unwired: 3 in]
            n193 = Concatenate Strings(w934, w926) -> (w936:string)
            n194 = Concatenate Strings(w935, w933, "\tLog Test" ("text"), w933, w936, "\n") -> (w928:string)
            n195 = Enqueue Element(queue=w929, element=w928, error in (no error)=w927) -> (error out=w925:errorcluster)  [unwired: 1 in, 2 out]
          }
        }
        n196 = Compound Arithmetic op=OR(w908, w907) -> (w906:bool)
        "S.L.B. Status" <- w906
        n197 = local read "Stop"() -> (w920:bool)
        n198 = Or(x=w906, y=w920) -> (x .or. y?=w919:bool)
      }
      n199 = while {
        shift-right: [w844] -> w157
        shift-left: w119 -> [w848]
        tunnel: w169 -> [w861]
        shift-right: [w850] -> w171
        shift-left: w172 -> [w852]
        shift-right: [w849] -> _
        shift-left: w173 -> [w851]
        shift-right: [w843] -> w160
        shift-left: w119 -> [w860]
        tunnel: [w842] -> w161
        stop <- w854 stop-if-true
        # "System log handler"
        n200 = call "Elapsed Time2"() -> ("Time has Elapsed"=w853:bool)  [unwired: 12 in, 7 out]
        n201 = Get Queue Status(queue=w861, error in (no error)=w860) -> (queue out=w846:refnum<queue>, error out=w845:errorcluster, # elements in queue=w859:i32)  [unwired: 1 in, 5 out]
        n202 = case shown="True" w853 {
          tunnel: w851 -> [w865 w868]
          tunnel: [w864 w869] -> w850
          tunnel: [w865 w868] -> w849
          tunnel: w852 -> [w864 _]
          tunnel: w848 -> [w863 w867]
          tunnel: [w863 w866] -> w847
          frame False {
          }
          frame True {
            n203 = call <vilib>:"Create File with Incrementing Suffix.vi"("error in (no error)"=w867, "file path"=w868) -> ("error out"=w866:errorcluster, "actual path"=w869:path)  [unwired: 7 in, 1 out]
          }
        }
        n204 = Wait (ms)(milliseconds to wait=u32 20) -> ()  [unwired: 1 out]
        n205 = Greater Or Equal?(x=w859, y=1) -> (x >= y?=w857:bool)
        n206 = case shown="True" w857 {
          tunnel: w847 -> [w872 w880]
          tunnel: w850 -> [_ w879]
          tunnel: [w872 w878] -> w844
          tunnel: w846 -> [w870 w877]
          tunnel: w845 -> [w871 w876]
          tunnel: [w871 w874] -> w843
          tunnel: [w870 w873] -> w842
          frame False {
          }
          frame True {
            n207 = Dequeue Element(queue=w877, error in (no error)=w876) -> (queue out=w873:refnum<queue>, element=w875:string, error out=w874:errorcluster)  [unwired: 1 in, 1 out]
            "System Log" <- w875
            n208 = call "txtfilewriter (SubVI).vi"("error in (no error)"=w880, "String"=w875, "actual path"=w879) -> ("error out"=w878:errorcluster)  [unwired: 8 in]
            "System Log Write Path" <- w879
          }
        }
        n209 = Compound Arithmetic op=OR(w843, w844) -> (w856:bool)
        "S.L.H. Status" <- w856
        n210 = local read "Stop"() -> (w855:bool)
        n211 = Or(x=w856, y=w855) -> (x .or. y?=w854:bool)
      }
      n212 = while {
        shift-right: [w442] -> w152
        shift-left: w119 -> [w454]
        tunnel: w141 -> [w445]
        tunnel: [w449] -> w165
        shift-right: [w441] -> w164
        shift-left: w119 -> [w444]
        stop <- w438 stop-if-true
        # "Message Sender"
        n213 = Get Queue Status(queue=w445, error in (no error)=w444) -> (queue out=w446:refnum<queue>, error out=w443:errorcluster, # elements in queue=w451:i32)  [unwired: 1 in, 5 out]
        n214 = Wait (ms)(milliseconds to wait=u32 20) -> ()  [unwired: 1 out]
        n215 = Greater Or Equal?(x=w451, y=1.0) -> (x >= y?=w447:bool)
        n216 = case shown="True" w447 {
          tunnel: w446 -> [w457 w463]
          tunnel: w443 -> [w456 w462]
          tunnel: [FALSE w461] -> w450
          tunnel: [w457 w460] -> w449
          tunnel: [_ w458] -> w448
          tunnel: [w456 w459] -> w441
          frame False {
          }
          frame True {
            n217 = Dequeue Element(queue=w463, error in (no error)=w462) -> (queue out=w460:refnum<queue>, element=w458:string, error out=w459:errorcluster)  [unwired: 1 in, 1 out]
            "Message to Send" <- w458
            n218 = String Length(string=w458) -> (length=w465:i32)
            n219 = Greater Or Equal?(x=w465, y=1) -> (x >= y?=w461:bool)
          }
        }
        n220 = case shown="True" w450 {
          tunnel: w448 -> [_ w547]
          tunnel: w454 -> [w470 w545]
          tunnel: [w468 w542] -> w442
          frame False {
            w466 = FALSE
            n221 = xnode "Digital output (1 sample) 2"("A/DIO0 (Pin 11)"=w466, "error in (no error)"=w470) -> ("error out"=w469:errorcluster)
            n222 = local write "LinkIt Response\nTimed Out 1"(w466) -> ()
            n223 = local write "LinkIt Response\nTimed Out 2"(w466) -> ()
            n224 = xnode "Digital input (1 sample) 3"("error in (no error)"=w469) -> ("A/DIO1 (Pin 13)"=w467:bool, "error out"=w468:errorcluster)
            n225 = local write "Pin 13 State"(w467) -> ()
            "Pin 11 State" <- w466
          }
          frame True {
            n226 = flat-sequence {
              tunnel: w547 -> [w552]
              tunnel: [w552] -> w548
              tunnel: TRUE -> [w549]
              tunnel: w545 -> [w551]
              tunnel: [w550] -> w544
              tunnel: w548 -> [w592]
              tunnel: w544 -> [w591]
              tunnel: [w589] -> w543
              tunnel: [w588] -> w541
              tunnel: w543 -> [w660]
              tunnel: [w658] -> w542
              tunnel: w541 -> [w654]
              frame #0 {
                n227 = xnode "Digital output (1 sample)"("A/DIO0 (Pin 11)"=w549, "error in (no error)"=w551) -> ("error out"=w550:errorcluster)
                n228 = local write "Pin 11 State"(w549) -> ()
              }
              frame #1 {
                n229 = while {
                  tunnel: w592 -> [w602]
                  tunnel: [w602] -> w593
                  shift-right: [w600] -> w590
                  shift-left: w591 -> [w599]
                  tunnel: [w594] -> w588
                  stop <- w596 stop-if-true
                  # "Wait for response"
                  n230 = call "Elapsed Time3"("error in (no error)"=w599) -> ("Elapsed Time (s)"=→"time to \nrespond":dbl, "Time has Elapsed"=w594:bool, "error out"=w598:errorcluster)  [unwired: 11 in, 5 out]
                  "LinkIt Response\nTimed Out 1" <- w594
                  n231 = Wait (ms)(milliseconds to wait=u32 1) -> ()  [unwired: 1 out]
                  n232 = xnode "Digital input (1 sample)"("error in (no error)"=w598) -> ("A/DIO1 (Pin 13)"=w597:bool, "error out"=w600:errorcluster)
                  "Pin 13 State" <- w597
                  n233 = Or(x=w597, y=w594) -> (x .or. y?=w596:bool)
                }
                n234 = xnode "UART 2"("Characters to Write"=w593, "error in (no error)"=w590) -> ("error out"=w589:errorcluster)  [unwired: 1 out]
              }
              frame #2 {
                w657 = FALSE ("A/DIO0 (Pin 11)")
                n235 = while {
                  shift-right: [w702] -> w659
                  shift-left: w660 -> [w703]
                  tunnel: [w696] -> w655
                  stop <- w700 stop-if-true
                  # "Wait for responce"
                  n236 = call "Elapsed Time4"("error in (no error)"=w703) -> ("Elapsed Time (s)"=→"Time to Send \nMessage":dbl, "Time has Elapsed"=w696:bool, "error out"=w699:errorcluster)  [unwired: 11 in, 5 out]
                  "LinkIt Response\nTimed Out 2" <- w696
                  n237 = Wait (ms)(milliseconds to wait=u32 1) -> ()  [unwired: 1 out]
                  n238 = xnode "Digital input (1 sample) 2"("error in (no error)"=w699) -> ("A/DIO1 (Pin 13)"=w697:bool, "error out"=w702:errorcluster)
                  n239 = Not(x=w697) -> (.not. x?=w701:bool)
                  n240 = local write "Pin 13 State"(w697) -> ()
                  n241 = Or(x=w701, y=w696) -> (x .or. y?=w700:bool)
                }
                n242 = Or(x=w655, y=w654) -> (x .or. y?=→"LinkIt Response\nTimed Out 3":bool)
                n243 = xnode "Digital output (1 sample) 3"("A/DIO0 (Pin 11)"=w657, "error in (no error)"=w659) -> ("error out"=w658:errorcluster)
                n244 = local write "Pin 11 State"(w657) -> ()
              }
            }
          }
        }
        n245 = local read "Stop"() -> (w439:bool)
        n246 = Compound Arithmetic op=OR(w441, w442) -> (w440:bool)
        "M.S. Status" <- w440
        n247 = Or(x=w440, y=w439) -> (x .or. y?=w438:bool)
      }
      n248 = while {
        stop <- w1051 stop-if-true
        # "Main Loop"
        n249 = local read "Initialisation \nsuccessfull"() -> (w1054:bool)
        n250 = local read "D.L.H. Status"() -> (w1057:bool)
        n251 = local read "S.L.H. Status"() -> (w1056:bool)
        n252 = local read "D.L.B. Status"() -> (w1048:bool)
        n253 = local read "S.L.B. Status"() -> (w1047:bool)
        n254 = local read "M.H. Status"() -> (w1053:bool)
        n255 = Wait (ms)(milliseconds to wait=u32 10) -> ()  [unwired: 1 out]
        n256 = Compound Arithmetic op=OR(w1048, w1047, w1053) -> (→"Data Queue Error":bool)
        n257 = Or(x=w1057, y=w1056) -> (x .or. y?=→"Storage Device Failure":bool)
        n258 = Not(x=w1054) -> (.not. x?=w1049:bool)
        n259 = Compound Arithmetic op=OR(w1049, w1057, w1048) -> (w1050:bool)
        n260 = local read "M.R. Status"() -> (w1044:bool)
        n261 = local read "M.S. Status"() -> (w1043:bool)
        n262 = Or(x="Stop", y=w1050) -> (x .or. y?=w1051:bool)
        n263 = local write "Stop"(w1051) -> ()
        n264 = Or(x=w1044, y=w1043) -> (x .or. y?=→"LinkIt Failure":bool)
        n265 = Not(x=w1044) -> (.not. x?=w1045:bool)
        n266 = And(x=w1045, y=w1043) -> (x .and. y?=→"DIO Failure":bool)
      }
      n267 = Release Queue(queue=w168, error in (no error)=w167) -> (error out=w159:errorcluster)  [unwired: 1 in, 2 out]
      n268 = Merge Errors(w158, w159) -> (w134:errorcluster)
      n269 = Release Queue(queue=w162, error in (no error)=w163) -> (error out=w155:errorcluster)  [unwired: 1 in, 2 out]
      n270 = Merge Errors(w151, w150, w149) -> (w138:errorcluster)
      n271 = Merge Errors(w142, w143, w148) -> (w136:errorcluster)
      n272 = Merge Errors(w155, w154) -> (w135:errorcluster)
      n273 = Release Queue(queue=w145, error in (no error)=w146) -> (error out=w140:errorcluster)  [unwired: 1 in, 2 out]
      n274 = Merge Errors(w147, w140) -> (w137:errorcluster)
      n275 = Release Queue(queue=w161, error in (no error)=w160) -> (error out=w156:errorcluster)  [unwired: 1 in, 2 out]
      n276 = Merge Errors(w156, w157) -> (w133:errorcluster)
      n277 = while {
        shift-right: [w1037] -> _
        shift-left: w179 -> [w1037]
        tunnel: [w1018] -> w180
        stop <- w1040 stop-if-true
        w1022 = ":" ("string")
        w1028 = 1
        # "method for calculating the uptime for the device measured in MM:DD:HH:MM:SS"
        # "System uptime"
        n278 = Get Date/Time In Seconds() -> (seconds since 1Jan1904=w1041:timestamp)
        n279 = Wait (ms)(milliseconds to wait=u32 100) -> ()  [unwired: 1 out]
        n280 = Subtract(x=w1041, y=w1037) -> (x-y=w1039:dbl)
        n281 = To Time Stamp(1:w1039) -> (0:w1021:timestamp)
        n282 = Get Date/Time String(seconds (now)=w1021, want seconds? (F)=TRUE) -> (date string=w1036:string)  [unwired: 1 in, 1 out]
        n283 = Match Pattern(string=w1036, regular expression="/04") -> (before substring=w1034:string)  [unwired: 1 in, 3 out]
        n284 = Match Pattern(string=w1034, regular expression="/") -> (before substring=w1032:string, after substring=w1031:string)  [unwired: 1 in, 2 out]
        n285 = Decimal String To Number(string=w1032) -> (number=w1030:i32)  [unwired: 2 in, 1 out]
        n286 = Decimal String To Number(string=w1031) -> (number=w1029:i32)  [unwired: 2 in, 1 out]
        n287 = Subtract(x=w1030, y=w1028) -> (x-y=w1026:i32)
        n288 = Subtract(x=w1029, y=w1028) -> (x-y=w1027:i32)
        n289 = Number To Decimal String(number=w1026) -> (decimal integer string=w1025:string)  [unwired: 1 in]
        n290 = Number To Decimal String(number=w1027) -> (decimal integer string=w1024:string)  [unwired: 1 in]
        n291 = Format Date/Time String(time format string (%c)="%H:%M:%S", seconds (now)=w1021) -> (date/time string=w1019:string)  [unwired: 1 in]
        n292 = Concatenate Strings(w1025, w1022, w1024, w1022, w1019) -> (w1018:string)
        "System Uptime" <- w1018
        n293 = local read "Stop"() -> (w1040:bool)
      }
      n294 = Release Queue(queue=w165, error in (no error)=w164) -> (error out=w153:errorcluster)  [unwired: 1 in, 2 out]
      n295 = Merge Errors(w153, w152) -> (w132:errorcluster)
      n296 = xnode "Invoke Method"("FPGA VI Reference In"=w124, "error in"=w125) -> ("FPGA VI Reference Out"=w126:refnum<k20>, "error out"=w127:errorcluster)
      n297 = Release Queue(queue=w128, error in (no error)=w129) -> (error out=w117:errorcluster)  [unwired: 1 in, 2 out]
      n298 = xnode "Close FPGA VI Reference"("FPGA VI Reference In"=w126, "error in"=w127) -> ("error out"=w116:errorcluster)
      n299 = Merge Errors(w117, w116, w139, w138, w137, w136, w135, w119, w134, w133, w132) -> (w130:errorcluster)
    }
    frame #2 {
      # "Close"
      n300 = call <vilib>:"Reset myRIO.vi"("error in (no error)"=w1061) -> ("error out"=w1063:errorcluster)  [unwired: 10 in]
      n301 = Unbundle By Name(w1063) -> ("status"=w1067:bool, "code"=w1066:i32, "source"=w1065:string)
      n302 = case shown="True" w1067 {
        tunnel: w1061 -> [w1068 w1090]
        tunnel: [w1068 w1088] -> w1060
        tunnel: w1066 -> [_ w1077]
        tunnel: w1065 -> [_ w1074]
        tunnel: w1062 -> [_ w1071]
        tunnel: w1064 -> [_ w1070]
        frame False {
        }
        frame True {
          w1075 = "\n"
          w1081 = "\t"
          # "logs errors to the current log file"
          # "error logger"
          n303 = Number To Decimal String(number=w1077) -> (decimal integer string=w1078:string)  [unwired: 1 in]
          n304 = Number To Decimal String(number=0) -> (decimal integer string=w1084:string)  [unwired: 1 in]
          n305 = Concatenate Strings("loop ", w1084) -> (w1082:string)
          n306 = Concatenate Strings("ERROR ", w1078, "\r", w1074) -> (w1076:string)
          n307 = Open/Create/Replace File(file path (use dialog)=w1071, error in=w1090, operation (0:open)=T12."open or create") -> (refnum out=w1093:refnum<file>, error out=w1094:errorcluster)  [unwired: 3 in, 1 out]
          n308 = Format Date/Time String() -> (date/time string=w1086:string)  [unwired: 3 in]
          n309 = Concatenate Strings(w1086, w1081, "\tLog Test" ("text"), w1081, w1082, w1081, w1075, w1076, w1075, "uptime" ("string"), w1070) -> (w1087:string)
          n310 = Set File Position(refnum=w1093, from (0:start)=enum16{"start", "end", "current"}."end", error in=w1094) -> (refnum out=w1096:refnum<file>, error out=w1095:errorcluster)  [unwired: 1 in]
          n311 = Write to Text File(file (use dialog)=w1096, text=w1087, error in=w1095) -> (refnum out=w1089:refnum<file>, error out=w1072:errorcluster)  [unwired: 1 in, 1 out]
          n312 = Close File(refnum=w1089, error in=w1072) -> (error out=w1088:errorcluster)  [unwired: 1 out]
        }
      }
      "error out" <- w1060
    }
  }
